vi "bsearch11.vi"(5 "val":i16, 7 "Array":i16[](array[numeric])) -> (0 "a":i32, 2 "idx":i32)   [LabVIEW 2010]
panel:
  # "индекс\nнайденного"
  # "индекс для\nвставки"
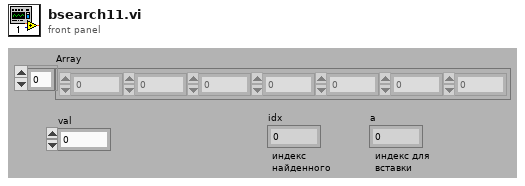
[diagram p1: front panel]
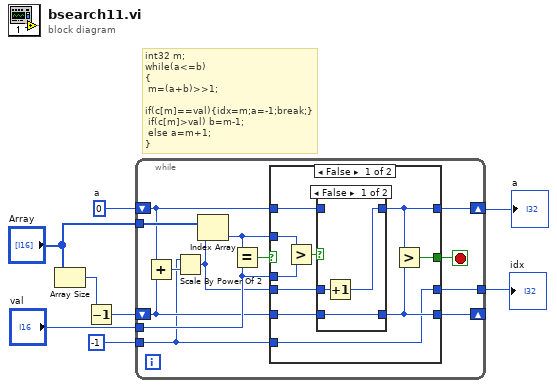
[diagram p0: block diagram]
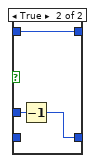
[diagram p2: hidden frame]
diagram:
  w3 = 0  # a
  # "int32 m;\nwhile(a<=b)\n{\n m=(a+b)>>1;\n if(c[m]==val){idx=m;a=-1;break;}\n if(c[m]>val) b=m-1;\n else a=m+1;\n}"
  n1 = Array Size(array="Array") -> (size(s)=w6:i32)
  n2 = Decrement(x=w6) -> (x-1=w1:i32)
  n3 = while {
    shift-right: [w15] -> w7
    shift-left: w3 -> [w17]
    shift-right: [w14] -> _
    shift-left: w1 -> [w16]
    tunnel: "Array" -> [w20]
    tunnel: "val" -> [w18]
    tunnel: -1 ("n") -> [w12]
    tunnel: [w9] -> w8
    stop <- w10 stop-if-true
    n4 = Add(x=w17, y=w16) -> (x+y=w21:i32)
    n5 = Scale By Power Of 2(n=w12, x=w21) -> (x*2^n=w13:i32)
    n6 = Index Array(array=w20, index=w13) -> (element=w19:i16)
    n7 = Equal?(x=w19, y=w18) -> (x = y?=w11:bool)
    n8 = case shown="False" w11 {
      selector: w11 -> [_ w41]
      tunnel: w19 -> [w31 _]
      tunnel: w18 -> [w30 _]
      tunnel: w17 -> [w28 _]
      tunnel: w16 -> [w27 w38]
      tunnel: [w26 w40] -> w15
      tunnel: [w25 w38] -> w14
      tunnel: [w23 w41] -> w10
      tunnel: w13 -> [w24 w39]
      tunnel: w12 -> [w22 w40]
      tunnel: [w22 w39] -> w9
      frame False {
        n9 = Greater?(x=w31, y=w30) -> (0:w29:bool)
        n10 = case shown="False" w29 {
          tunnel: [w32 w37] -> w26
          tunnel: w28 -> [_ w37]
          tunnel: [w34 w36] -> w25
          tunnel: w24 -> [w33 w35]
          tunnel: w27 -> [w34 _]
          frame False {
            n11 = Increment(x=w33) -> (x+1=w32:i32)
          }
          frame True {
            n12 = Decrement(x=w35) -> (x-1=w36:i32)
          }
        }
        n13 = Greater?(x=w26, y=w25) -> (0:w23:bool)
      }
      frame True {
      }
    }
  }
  "idx" <- w8
  "a" <- w7
